vi "TDMSlogg_Init.vi"(0 "object in":refnum<class "TDMSlogg.lvclass">, 2 "Folder path":path, 5 "error in (no error)":errorcluster) -> (14 "object out":refnum<class "TDMSlogg.lvclass">, 19 "error out":errorcluster)   [LabVIEW 2019, in "TDMSlogg.lvclass"]
uses:
  TDMSlogg.lvclass
  TDMSlogg.lvclass/TDMSlogg.ctl
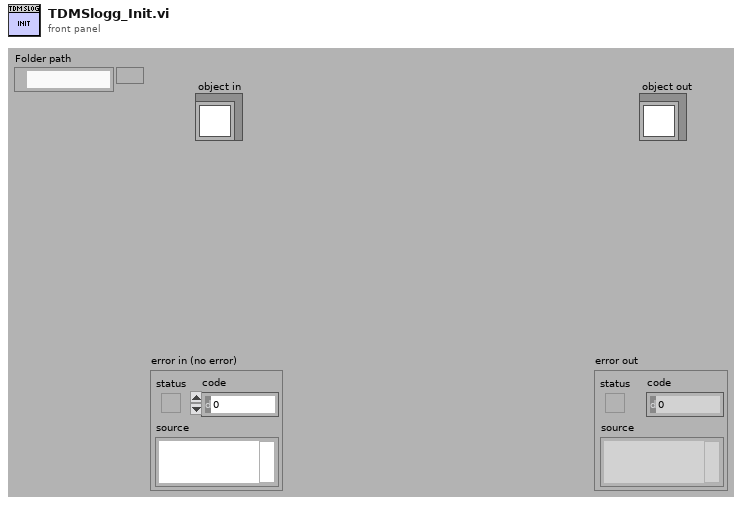
[diagram p1: front panel]
types:
  T1 = enum16{"open", "open or create", "create or replace", "create", "open (read-only)"}
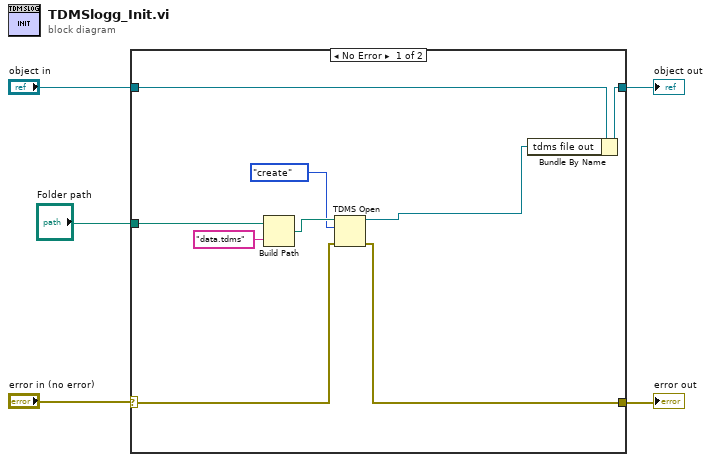
[diagram p0: block diagram]
diagram:
  n1 = case shown="No Error" "error in (no error)" {
    selector: "error in (no error)" -> [w8 w15]
    tunnel: "object in" -> [w14 w16]
    tunnel: [w13 w16] -> w4
    tunnel: [w7 w15] -> w2
    tunnel: "Folder path" -> [w10 _]
    frame No Error {
      n2 = Build Path(base path=w10, name or relative path="data.tdms") -> (appended path=w12:path)
      n3 = TDMS Open(8:w8, 10:T1."create" ("operation (0:open)"), 11:w12) -> (0:w7:errorcluster, 3:w6:refnum<k34>)  [unwired: 4 in]
      n4 = Bundle By Name(cluster=w14, "tdms file out"=w6) -> (w13:refnum<class "TDMSlogg.lvclass">)
    }
    frame Error {
    }
  }
  "object out" <- w4
  "error out" <- w2
